vi "log file viewer.vi"() -> ()   [LabVIEW 2020]
uses:
  <vilib>/Utility/sysdir.llb/System Directory Type.ctl
  <vilib>/addons/_JKI Toolkits/State Machine/_JKI_lib_State_Machine.llb/Select State(s)_err__jki_lib_state_machine.vi
  <vilib>/regexp/Match Regular Expression.xnode
  <vilib>/JDP Science/JSONtext/JSONtext.lvlib
panel:
  in  "Open File":bool
  in  "refresh":bool
  in  "Log Files":i32(listbox)
  out "message":string
  in  "timestamp":i32(listbox)
  in  "Exit":bool
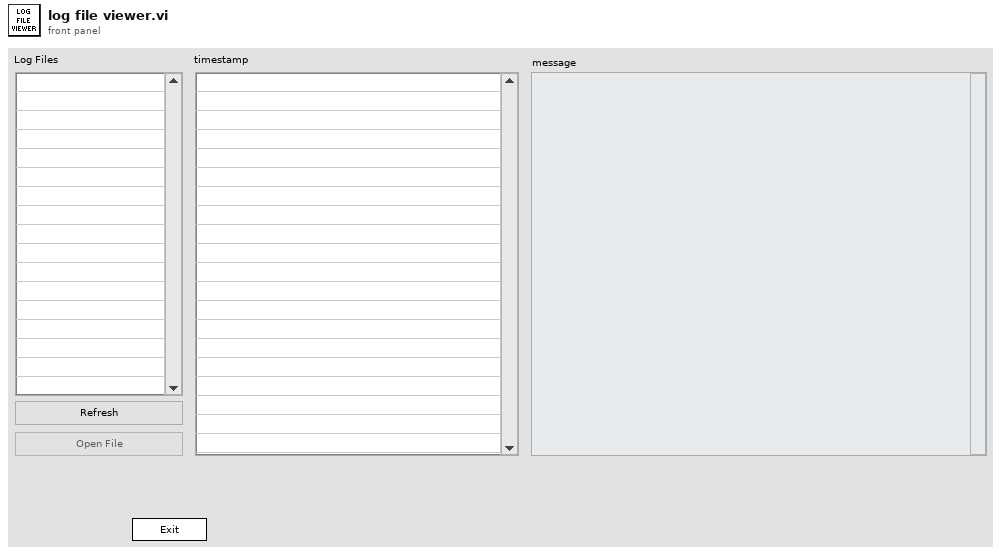
[diagram p1: front panel]
types:
  T1 = enum8{"Enabled", "Disabled", "Disabled and Grayed Out"}
  T2 = enum32{"Invalid", "Standard", "Closed", "Hidden", "Minimized", "Maximized"}
  T3 = enum32{"invalid app kind", "Development System", "Run Time System", "Student Edition", "Embedded LabVIEW", "Evaluation", "Custom"}
  T4 = cluster{"Core":cluster{"Current VI Reference":refnum<vi>, "Close Panel on Exit?":bool}, "log file":path, "elements":string[], "Log Directory":path}
  T5 = typedef "System Directory Type.ctl" = i32
  T6 = cluster{"Current VI Reference":refnum<vi>, "Close Panel on Exit?":bool}
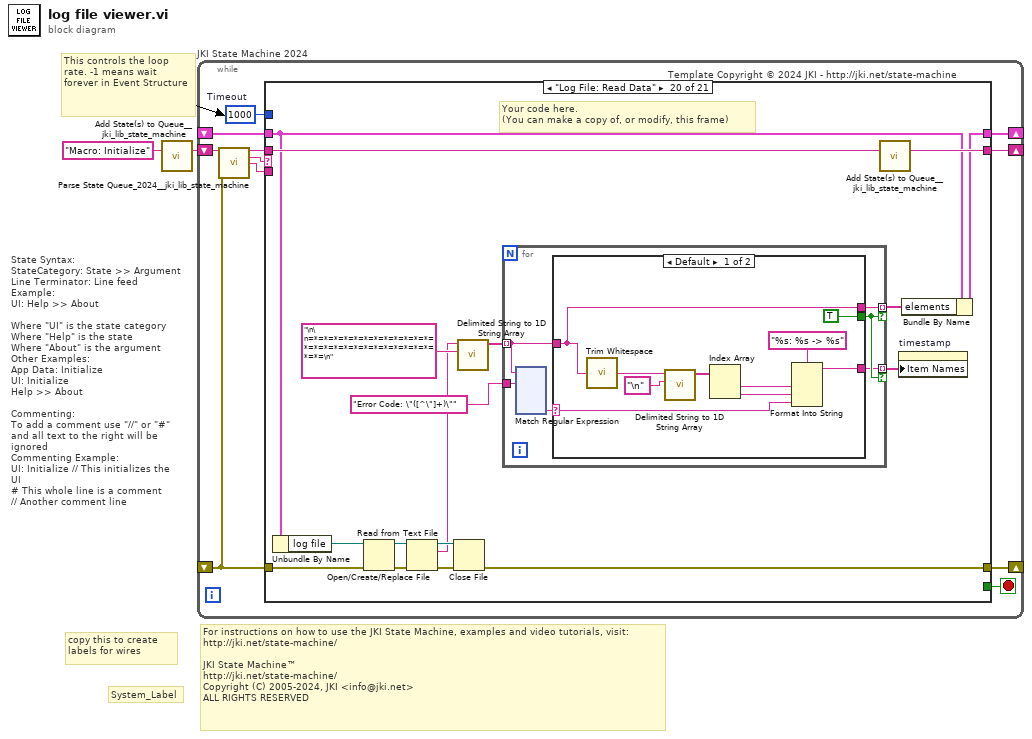
[diagram p0: block diagram]
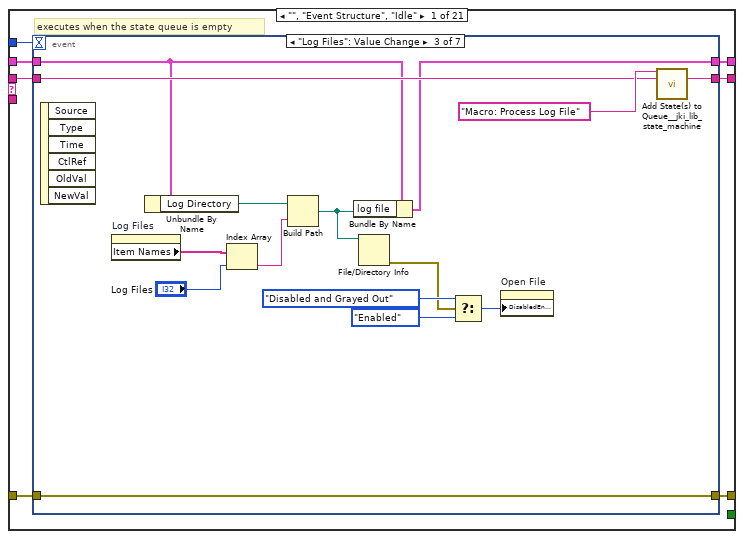
[diagram p2: hidden frame]
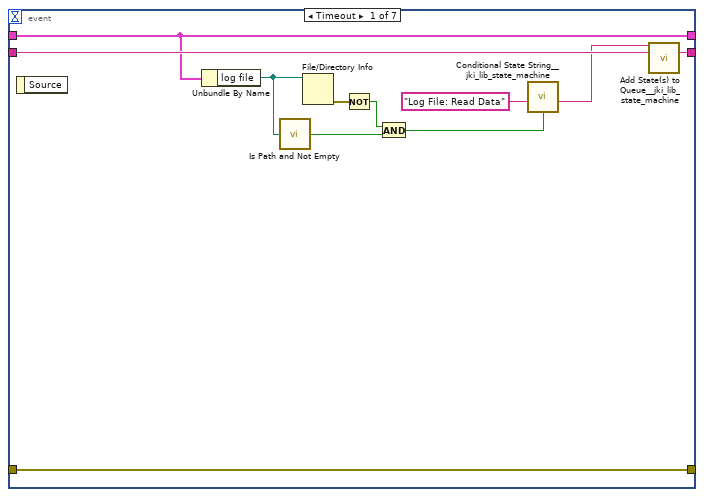
[diagram p3: hidden frame]
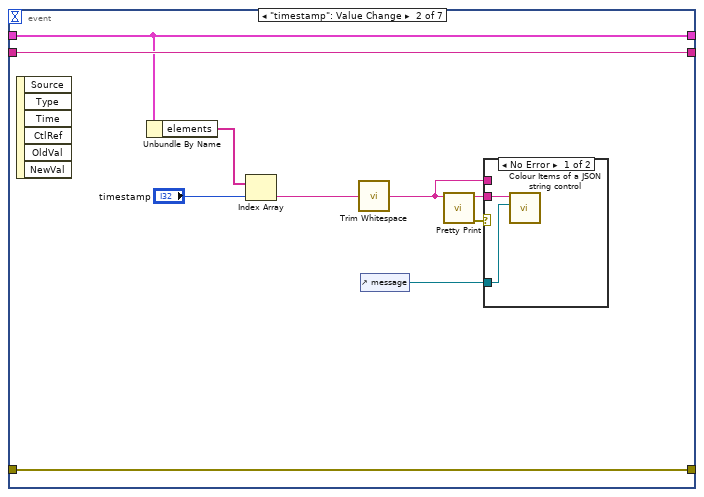
[diagram p4: hidden frame]
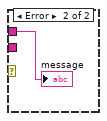
[diagram p5: hidden frame]
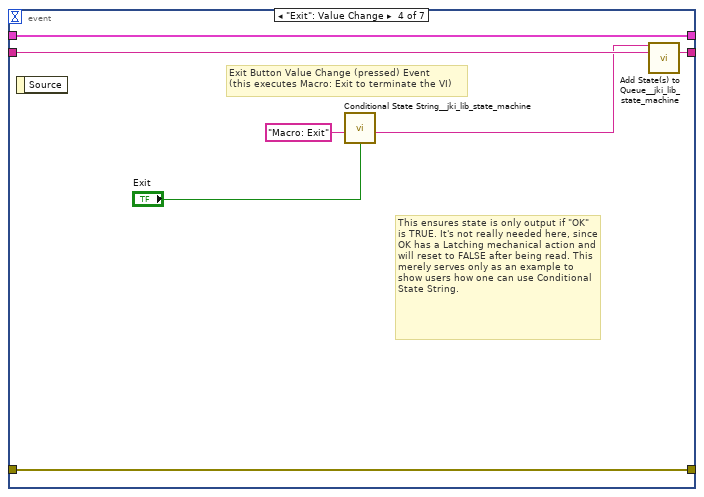
[diagram p6: hidden frame]
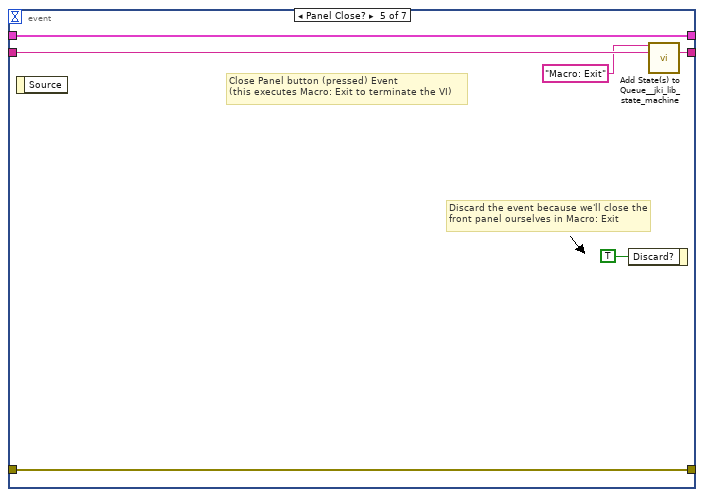
[diagram p7: hidden frame]
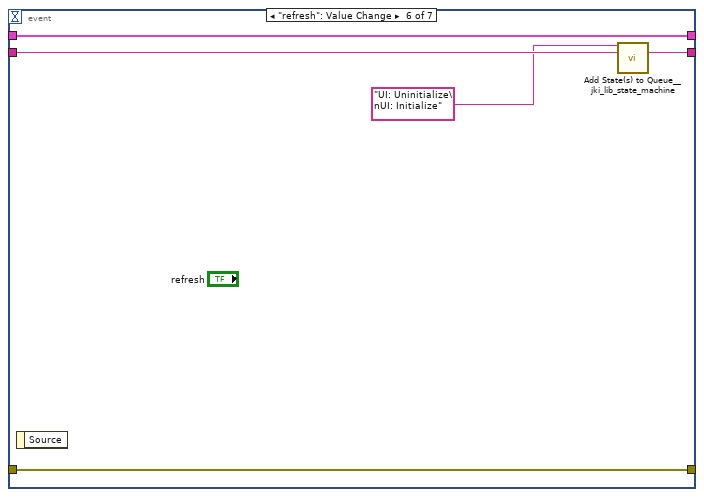
[diagram p8: hidden frame]
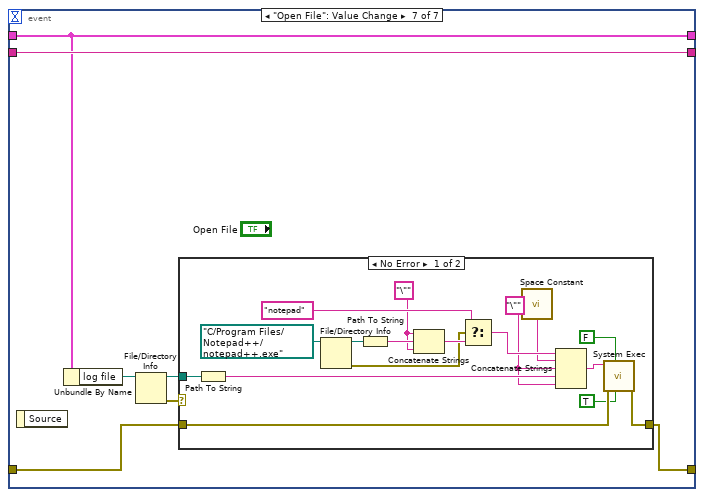
[diagram p9: hidden frame]
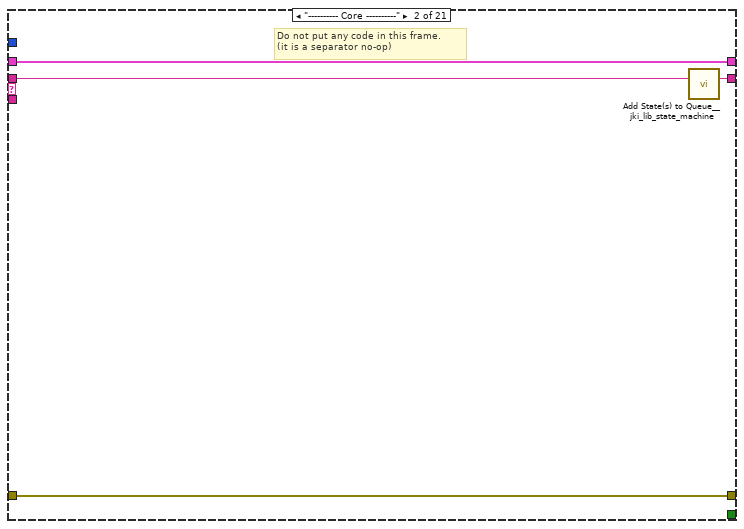
[diagram p11: hidden frame]
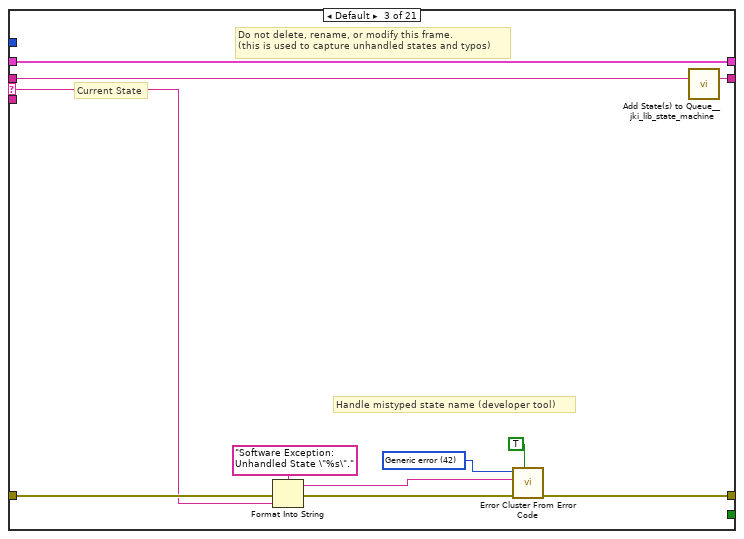
[diagram p12: hidden frame]
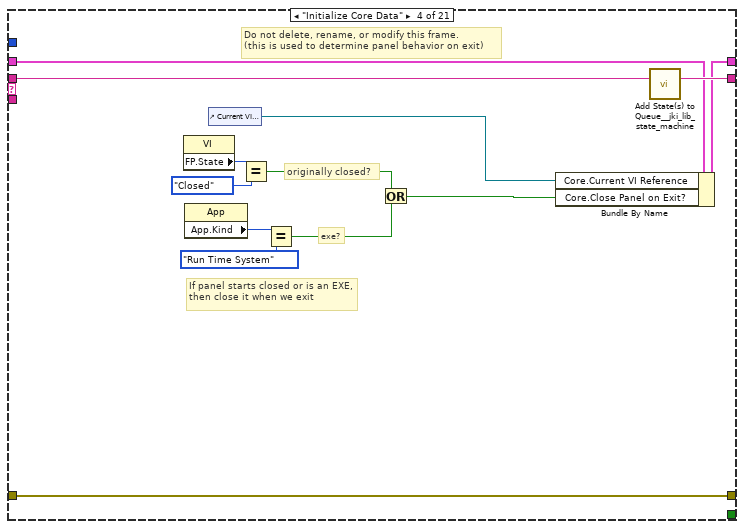
[diagram p13: hidden frame]
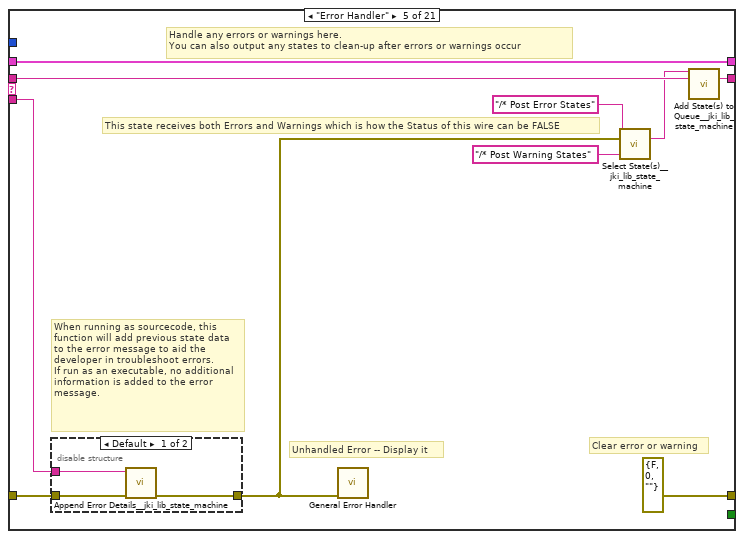
[diagram p14: hidden frame]
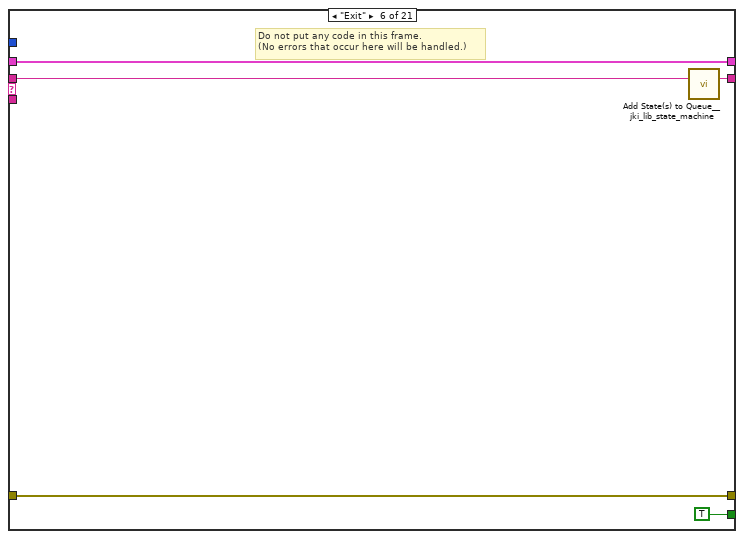
[diagram p16: hidden frame]
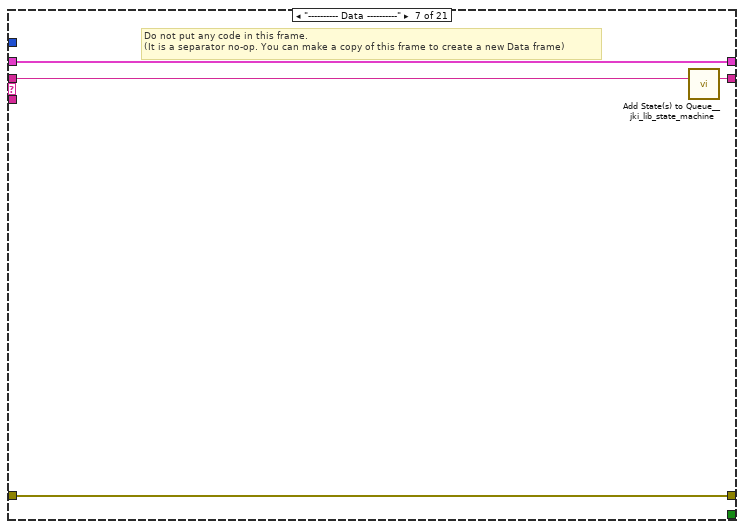
[diagram p17: hidden frame]
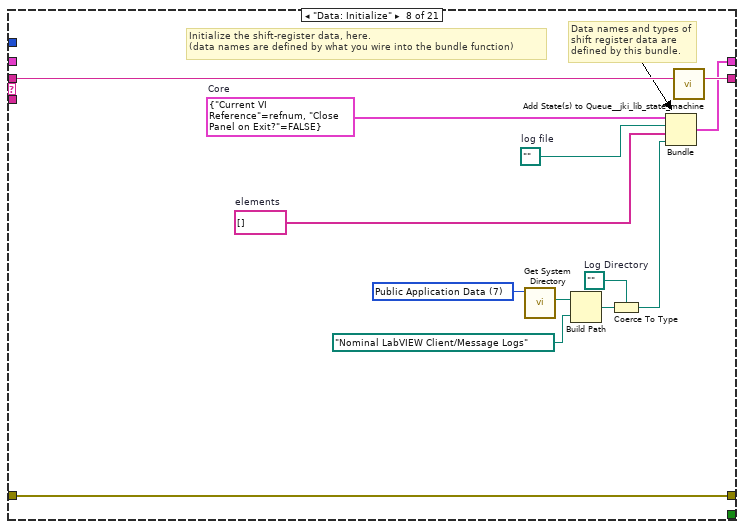
[diagram p18: hidden frame]
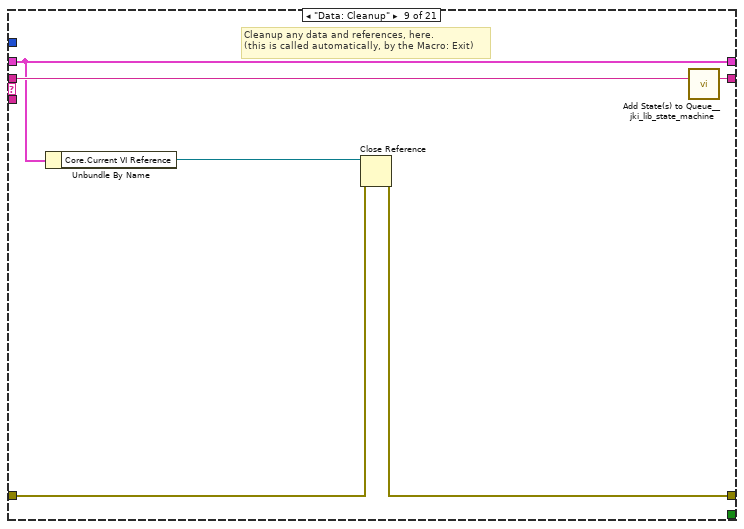
[diagram p19: hidden frame]
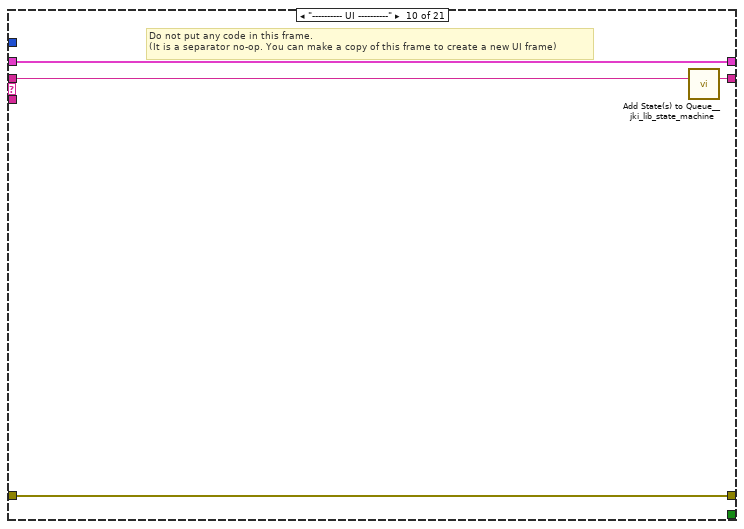
[diagram p20: hidden frame]
diagram:
  # "For instructions on how to use the JKI State Machine, examples and video tutorials, visit:\nhttp://jki.net/state-machine/\n\nJKI State Machine™\nhttp://jki.net/state-machine/\nCopyright (C) 2005-2024, JKI <info@jki.net>\nALL RIGHTS RESERVED"
  # "State Syntax:\nStateCategory: State >> Argument\nLine Terminator: Line feed\nExample:\nUI: Help >> About\n\nWhere \"UI\" is the state category\nWhere \"Help\" is the state\nWhere \"About\" is the argument\nOther Examples:\nApp Data: Initialize\nUI: Initialize\nHelp >> About\n\nCommenting:\nTo add a comment use \"//\" or \"#\" and all text to the right will be ignored\nCommenting Example:\nUI: Initialize // This initializes the UI\n# This whole line is a comment\n// Another comment line"
  # "copy this to create labels for wires"
  # "This controls the loop rate. -1 means wait forever in Event Structure"
  # "System_Label"
  n1 = call <vilib>:"Add State(s) to Queue__jki_lib_state_machine.vi"("State(s) in (\"\")"="Macro: Initialize") -> ("States Out"=w2:string)  [unwired: 14 in]
  n2 = while "JKI State Machine 2024" {
    shift-right: [w6] -> _
    shift-left: _ -> [w5]
    shift-right: [w9] -> _
    shift-left: _ -> [w3]
    shift-right: [w8] -> _
    shift-left: w2 -> [w10]
    stop <- w7 stop-if-true
    w4 = 1000  # Timeout
    # "Template Copyright © 2024 JKI - http://jki.net/state-machine"
    n3 = call <vilib>:"Parse State Queue_2024__jki_lib_state_machine.vi"("State Queue"=w10, "Error In (no error)"=w3) -> ("Remaining States"=w12:string, "Current State"=w13:string, "Arguments"=w11:string)  [unwired: 11 in]
    n4 = case shown="\"Log File: Read Data\"" w13 {
      selector: w13 -> [_ _ w107 _ _ _ _ _ _ _ _ _ _ _ _ _ _ _ _ _ _]
      tunnel: w12 -> [w20 w106 w111 w130 w140 w149 w153 w166 w172 w176 w184 w186 w197 w208 w277 w282 w291 w296 w300 w317 w466]
      tunnel: w11 -> [_ _ _ _ w135 _ _ _ _ _ _ _ w192 w202 _ _ _ _ _ _ _]
      tunnel: w5 -> [w18 w103 w109 w123 w137 w147 w150 _ w167 w173 w180 w190 w195 w204 w274 w279 w289 w294 w297 w304 w463]
      tunnel: [w17 w104 w113 w127 errorcluster {"status"=FALSE, "code"=0, "source"=""} ("error out") w146 w151 w163 w168 w174 w182 w189 w193 w205 w275 w280 w286 w293 w298 w310 w464] -> w9
      tunnel: w3 -> [w14 w104 w112 w127 w136 w146 w151 w163 w169 w174 w182 w189 w194 w206 w275 w280 w286 w293 w298 w309 w464]
      tunnel: [w19 w105 w110 w129 w139 w148 w152 w165 w171 w175 w183 w191 w196 w207 w276 w281 w290 w295 w299 w316 w465] -> w8
      tunnel: [_ _ _ _ _ TRUE _ _ _ _ _ _ _ _ _ _ _ _ _ _ _] -> w7
      tunnel: [w16 w103 w109 w128 w137 w147 w150 w164 w167 w173 w180 w190 w195 w204 w274 w279 w289 w294 w297 w303 w463] -> w6
      tunnel: w4 -> [w15 _ _ _ _ _ _ _ _ _ _ _ _ _ _ _ _ _ _ _ _]
      frame "", "Event Structure", "Idle" {
        # "executes when the state queue is empty"
        n5 = event shown="[2] \"Log Files\": Value Change" {
          selector: _ -> [_ _ _ _ _ _ _]
          dyn-events: _ -> [_ _ _ _ _ _ _]
          timeout: w15 -> [_ _ _ _ _ _ _]
          tunnel: w20 -> [w31 w41 w57 w66 w72 w75 w84]
          tunnel: [w30 w41 w56 w65 w71 w76 w84] -> w19
          tunnel: w18 -> [w28 w40 w51 w63 w69 w77 w83]
          tunnel: [w29 w33 w59 w64 w70 w74 w78] -> w17
          tunnel: w14 -> [w29 w33 w59 w64 w70 w74 w79]
          tunnel: [w28 w40 w50 w63 w69 w77 w83] -> w16
          event Timeout {
            n6 = event-data() -> ()  [unwired: 1 in, 1 out]
            n7 = Unbundle By Name(w28) -> ("log file"=w26:path)
            n8 = call <vilib>:"Is Path and Not Empty.vi"("path"=w26) -> ("Is Path and Not Empty?"=w25:bool)  [unwired: 4 in]
            n9 = File/Directory Info(path=w26) -> (error out=w27:errorcluster)  [unwired: 1 in, 6 out]
            n10 = Not(x=w27) -> (.not. x?=w24:bool)
            n11 = And(x=w24, y=w25) -> (x .and. y?=w22:bool)
            n12 = call <vilib>:"Conditional State String__jki_lib_state_machine.vi"("Do State(s)?"=w22, "State"="Log File: Read Data") -> ("State Out"=w23:string)  [unwired: 7 in]
            n13 = call <vilib>:"Add State(s) to Queue__jki_lib_state_machine.vi"("State(s) in Front (\"\")"=w23, "State(s) in (\"\")"=w31) -> ("States Out"=w30:string)  [unwired: 13 in]
          }
          event "timestamp": Value Change {
            n14 = event-data() -> ()  [unwired: 1 in, 6 out]
            n15 = Unbundle By Name(w40) -> ("elements"=w39:string[])
            n16 = Index Array(array=w39, index="timestamp") -> (element=w32:string)
            n17 = call <vilib>:"Trim Whitespace.vi"("string"=w32) -> ("trimmed string"=w34:string)  [unwired: 1 in]
            n18 = control-ref of="message"() -> (w37:refnum<vi>)
            n19 = call <vilib>:"Pretty Print.vi"("JSON"=w34) -> ("error out"=w35:errorcluster, "<JSON>"=w36:string)  [unwired: 8 in, 1 out]
            n20 = case shown="No Error" w35 {
              tunnel: w37 -> [w43 _]
              tunnel: w36 -> [w42 _]
              tunnel: w34 -> [_ w44]
              frame No Error {
                n21 = call <vilib>:"Colour Items of a JSON string control.vi"("String Control"=w43, "JSON"=w42) -> ()  [unwired: 9 in, 1 out]
              }
              frame Error {
                "message" <- w44
              }
            }
          }
          event "Log Files": Value Change {
            n22 = event-data() -> ()  [unwired: 1 in, 6 out]
            n23 = property on="Log Files" class="LstBox (strict)"() -> ("Item Names"=w54:string[])  [unwired: 2 in, 2 out]
            n24 = Unbundle By Name(w51) -> ("Log Directory"=w55:path)
            n25 = Index Array(array=w54, index="Log Files") -> (element=w52:string)
            n26 = Build Path(base path=w55, name or relative path=w52) -> (appended path=w46:path)
            n27 = Bundle By Name(cluster=w51, "log file"=w46) -> (w50:T4)
            n28 = File/Directory Info(path=w46) -> (error out=w45:errorcluster)  [unwired: 1 in, 6 out]
            n29 = Select(t=T1."Disabled and Grayed Out" ("Disabled"), s=w45, f=T1."Enabled" ("Disabled")) -> (s? t:f=w47:T1)
            n30 = property on="Open File" class="Bool"("DisabledEnum"=w47) -> ()  [unwired: 2 in, 2 out]
            n31 = call <vilib>:"Add State(s) to Queue__jki_lib_state_machine.vi"("State(s) in Front (\"\")"="Macro: Process Log File" ("string"), "State(s) in (\"\")"=w57) -> ("States Out"=w56:string)  [unwired: 13 in]
          }
          event "Exit": Value Change {
            # "This ensures state is only output if \"OK\" is TRUE. It's not really needed here, since OK has a Latching mechanical action and will reset to FALSE after being read. This merely serves only as an example to show users how one can use Conditional State String."
            # "Exit Button Value Change (pressed) Event\n(this executes Macro: Exit to terminate the VI)"
            n32 = event-data() -> ()  [unwired: 1 in, 1 out]
            n33 = call <vilib>:"Conditional State String__jki_lib_state_machine.vi"("Do State(s)?"="Exit", "State"="Macro: Exit") -> ("State Out"=w60:string)  [unwired: 7 in]
            n34 = call <vilib>:"Add State(s) to Queue__jki_lib_state_machine.vi"("State(s) in Front (\"\")"=w60, "State(s) in (\"\")"=w66) -> ("States Out"=w65:string)  [unwired: 13 in]
          }
          event Panel Close? {
            # "Discard the event because we'll close the front panel ourselves in Macro: Exit"
            # "Close Panel button (pressed) Event\n(this executes Macro: Exit to terminate the VI)"
            n35 = event-data() -> ()  [unwired: 1 in, 1 out]
            n36 = event-data("Discard?"=TRUE) -> ()  [unwired: 1 in, 1 out]
            n37 = call <vilib>:"Add State(s) to Queue__jki_lib_state_machine.vi"("State(s) in Front (\"\")"="Macro: Exit", "State(s) in (\"\")"=w72) -> ("States Out"=w71:string)  [unwired: 13 in]
          }
          event "refresh": Value Change {
            n38 = event-data() -> ()  [unwired: 1 in, 1 out]
            n39 = call <vilib>:"Add State(s) to Queue__jki_lib_state_machine.vi"("State(s) in Front (\"\")"="UI: Uninitialize\nUI: Initialize" ("State(s) in Front (\"\")"), "State(s) in (\"\")"=w75) -> ("States Out"=w76:string)  [unwired: 13 in]
          }
          event "Open File": Value Change {
            n40 = event-data() -> ()  [unwired: 1 in, 1 out]
            n41 = Unbundle By Name(w83) -> ("log file"=w82:path)
            n42 = File/Directory Info(path=w82) -> (path out=w80:path, error out=w81:errorcluster)  [unwired: 1 in, 5 out]
            n43 = case shown="No Error" w81 {
              tunnel: w80 -> [w98 _]
              tunnel: w79 -> [w92 w102]
              tunnel: [w91 w102] -> w78
              frame No Error {
                w88 = "\"" ("string")
                w95 = "\"" ("string")
                n44 = Path To String(path=w98) -> (string=w96:string)
                n45 = File/Directory Info(path=path "C:/Program Files/Notepad++/notepad++.exe") -> (path out=w101:path, error out=w86:errorcluster)  [unwired: 1 in, 5 out]
                n46 = Path To String(path=w101) -> (string=w89:string)
                n47 = Concatenate Strings(w88, w89, w88) -> (w87:string)
                n48 = Select(t="notepad", s=w86, f=w87) -> (s? t:f=w97:string)
                n49 = call <vilib>:"Space Constant.vi"() -> ("String"=w94:string)
                n50 = Concatenate Strings(w97, w94, w95, w96, w95) -> (w93:string)
                n51 = call <vilib>:"System Exec.vi"("run minimized? (F)"=TRUE, "wait until completion? (T)"=FALSE, "error in (no error)"=w92, "command line"=w93) -> ("error out"=w91:errorcluster)  [unwired: 4 in, 3 out]
              }
              frame Error {
              }
            }
          }
        }
      }
      frame "---------- Core ----------" {
        # "Do not put any code in this frame.\n(it is a separator no-op)"
        n52 = call <vilib>:"Add State(s) to Queue__jki_lib_state_machine.vi"("State(s) in (\"\")"=w106) -> ("States Out"=w105:string)  [unwired: 14 in]
      }
      frame Default {
        w116 = 42 items=["No error", "Argument error", "Memory is full", "Out of zone", "End of file", "File already open", "Generic file I/O error", "File not found", "File permission error", "Disk is full", "Duplicate path", "Too many files open", "System feature not enabled", "Resource file not found", "Cannot add resource", "Resource not found", "Image not found", "Image memory error", "Pen does not exist", "Config type invalid", "Config token not found", "Config parse error", "Config memory error", "Bad external code format", "Bad external code offset", "External code not present", "Null window", "Destroy window error", "Null menu", "Print aborted", "Bad print record", "Print driver error", "Windows error during printing", "Memory error during printing", "Print dialog error", "Generic print error", "Invalid device refnum", "Device not found", "Device parameter error", "Device unit error", "Cannot open device", "Device call aborted", "Generic error", "Cancelled by user", "Object ID too low", "Object ID too high", "Object not in heap", "Unknown heap", "Unknown object (invalid DefProc)", "Unknown object (DefProc not in table)", "Message out of range", "Invalid (null) method", "Unknown message", "Manager call not supported", "Bad address", "Network operation in progress", "Network operation timed out", "Connection is busy", "Network attribute not supported", "Network error", "Address in use", "System out of memory", "Connection aborted", "Connection refused", "Not connected", "Already connected", "Connection closed", "Initialization error (interapplication manager)", "Bad occurrence", "Wait on unbound occurrence handler", "Occurrence queue overflow", "Datalog type conflict", "Unused", "Unrecognized type (interapplication manager)", "Memory corrupt", "Failed to make temporary DLL", "Old CIN version", "Drag socket not found", "Failed to load drop-object", "Failed to register OLE object", "Failed to release OLE object", "Format specifier type mismatch", "Unknown format specifier", "Too few format specifiers", "Too many format specifiers", "Scan failed", "Newer CIN version", "Error converting to variant", "Runtime menu error", "Password tampered", "Variant attribute not found", "Incompatible variant data type", "Event data is not available", "Event Store is not present", "Occurrence is not found", "Event Queue is not created", "Event info is not available", "Refnum passed is NULL", "Error retrieving Class GUID", "Error retrieving CoClass GUID", "Error retrieving TypeLib GUID.", "Bad built application magic bytes.", "Specific driver is different from the specific driver associated with the Logical Name.", "There is no session opened to the class driver.", "Max Error", "MAX - Error with config objects", "MAX - Error loading configuration", "MAX - Group not supported"]
        # "Current State"
        # "Do not delete, rename, or modify this frame.\n(this is used to capture unhandled states and typos)"
        # "Handle mistyped state name (developer tool)"
        n53 = Format Into String(format string="Software Exception: Unhandled State \"%s\"." ("message"), error in=w112, w107) -> (resulting string=w115:string, error out=w114:errorcluster)  [unwired: 1 in]
        n54 = call <vilib>:"Error Cluster From Error Code.vi"("show call chain? (False)"=TRUE, "error in (no error)"=w114, "error message (\"\")"=w115, "error code (0)"=w116) -> ("error out"=w113:errorcluster)  [unwired: 5 in]
        n55 = call <vilib>:"Add State(s) to Queue__jki_lib_state_machine.vi"("State(s) in (\"\")"=w111) -> ("States Out"=w110:string)  [unwired: 14 in]
      }
      frame "Initialize Core Data" {
        # "Do not delete, rename, or modify this frame.\n(this is used to determine panel behavior on exit)"
        # "originally closed?"
        # "exe?"
        # "If panel starts closed or is an EXE, then close it when we exit"
        n56 = property class="VI"() -> ("FP.State"=w120:T2)  [unwired: 2 in, 2 out]
        n57 = property class="App"() -> ("App.Kind"=w126:T3)  [unwired: 2 in, 2 out]
        n58 = control-ref of="Current VI Reference"() -> (w121:refnum<vi>)
        n59 = Equal?(x=w120, y=T2."Closed" ("Front Panel Window:State")) -> (x = y?=w118:bool)
        n60 = Equal?(x=w126, y=T3."Run Time System" ("Application:Kind")) -> (x = y?=w124:bool)
        n61 = Or(x=w118, y=w124) -> (x .or. y?=w122:bool)
        n62 = Bundle By Name(cluster=w123, "Core.Current VI Reference"=w121, "Core.Close Panel on Exit?"=w122) -> (w128:T4)
        n63 = call <vilib>:"Add State(s) to Queue__jki_lib_state_machine.vi"("State(s) in (\"\")"=w130) -> ("States Out"=w129:string)  [unwired: 14 in]
      }
      frame "Error Handler" {
        # "When running as sourcecode, this function will add previous state data to the error message to aid the developer in troubleshoot errors.\nIf run as an executable, no additional information is added to the error message."
        # "This state receives both Errors and Warnings which is how the Status of this wire can be FALSE"
        # "Unhandled Error -- Display it"
        # "Handle any errors or warnings here.\nYou can also output any states to clean-up after errors or warnings occur"
        # "Clear error or warning"
        n64 = disable-structure shown="Default" {
          disable-tunnel: w136 -> [w143 w144]
          disable-tunnel: w135 -> [w142 _]
          disable-tunnel: [w141 w144] -> w134
          frame condition #0 (active) {
            n65 = call <vilib>:"Append Error Details__jki_lib_state_machine.vi"("error in (no error)"=w143, "Previous State and Argument(s)"=w142) -> ("error out"=w141:errorcluster)  [unwired: 9 in]
          }
          frame condition #1 {
          }
        }
        n66 = call <vilib>:"General Error Handler.vi"("error in (no error)"=w134) -> ()  [unwired: 10 in, 5 out]
        n67 = call-poly <vilib>:"Select State(s)__jki_lib_state_machine.vi"("State(s) if True (\"\")"="/* Post Error States", "Select"=w134, "State(s) if False (\"\")"="/* Post Warning States") -> ("States Out"=w132:string)  [unwired: 12 in]
        n68 = call <vilib>:"Add State(s) to Queue__jki_lib_state_machine.vi"("State(s) in Front (\"\")"=w132, "State(s) in (\"\")"=w140) -> ("States Out"=w139:string)  [unwired: 13 in]
      }
      frame "Exit" {
        # "Do not put any code in this frame.\n(No errors that occur here will be handled.)"
        n69 = call <vilib>:"Add State(s) to Queue__jki_lib_state_machine.vi"("State(s) in (\"\")"=w149) -> ("States Out"=w148:string)  [unwired: 14 in]
      }
      frame "---------- Data ----------" {
        # "Do not put any code in this frame.\n(It is a separator no-op. You can make a copy of this frame to create a new Data frame)"
        n70 = call <vilib>:"Add State(s) to Queue__jki_lib_state_machine.vi"("State(s) in (\"\")"=w153) -> ("States Out"=w152:string)  [unwired: 14 in]
      }
      frame "Data: Initialize" {
        w154 = path ""  # Log Directory
        w159 = T5 7 items=["User Home"=0, "User Desktop"=1, "User Documents"=2, "User Application Data"=3, "User Preferences"=4, "User Temporary"=5, "Public Documents"=6, "Public Application Data"=7, "Public Preferences"=8, "Public Cache"=13, "System Core Libraries"=9, "System Installed Libraries"=10, "Application Files"=11, "Boot Volume Root"=12] ("system directory type")
        w160 = string[] []  # elements
        w161 = path ""  # log file
        w162 = T6 {"Current VI Reference"=refnum, "Close Panel on Exit?"=FALSE}  # Core
        # "Data names and types of shift register data are defined by this bundle."
        # "Initialize the shift-register data, here.\n(data names are defined by what you wire into the bundle function)"
        n71 = call <vilib>:"Get System Directory.vi"("system directory type"=w159) -> ("system directory"=w158:path)  [unwired: 10 in]
        n72 = Build Path(base path=w158, name or relative path=path "Nominal LabVIEW Client/Message Logs") -> (appended path=w156:path)
        n73 = Coerce To Type(0:w156, 1:w154) -> (2:w155:path)
        n74 = Bundle("Core"=w162, "log file"=w161, "elements"=w160, "Log Directory"=w155) -> (w164:T4)  [unwired: 1 in]
        n75 = call <vilib>:"Add State(s) to Queue__jki_lib_state_machine.vi"("State(s) in (\"\")"=w166) -> ("States Out"=w165:string)  [unwired: 14 in]
      }
      frame "Data: Cleanup" {
        # "Cleanup any data and references, here.\n(this is called automatically, by the Macro: Exit)"
        n76 = Unbundle By Name(w167) -> ("Core.Current VI Reference"=w170:refnum<vi>)
        n77 = Close Reference(reference=w170, error in (no error)=w169) -> (error out=w168:errorcluster)
        n78 = call <vilib>:"Add State(s) to Queue__jki_lib_state_machine.vi"("State(s) in (\"\")"=w172) -> ("States Out"=w171:string)  [unwired: 14 in]
      }
      frame "---------- UI ----------" {
        # "Do not put any code in this frame.\n(It is a separator no-op. You can make a copy of this frame to create a new UI frame)"
        n79 = call <vilib>:"Add State(s) to Queue__jki_lib_state_machine.vi"("State(s) in (\"\")"=w176) -> ("States Out"=w175:string)  [unwired: 14 in]
      }
      frame "UI: Initialize" {
        w178 = 0 ("Top Row")
        # "Initialize the User Interface, here.\n(this is called automatically, by the Macro: Initialize)"
        n80 = Unbundle By Name(w180) -> ("Log Directory"=w179:path)
        n81 = List Folder(path=w179) -> (filenames=w181:string[])  [unwired: 3 in, 3 out]
        n82 = property on="Open File" class="Bool"("DisabledEnum"=T1."Disabled and Grayed Out" ("Disabled")) -> ()  [unwired: 2 in, 2 out]
        n83 = property on="Log Files" class="LstBox (strict)"("Item Names"=w181, "Top Row"=w178) -> ()  [unwired: 2 in, 2 out]
        n84 = property on="timestamp" class="LstBox (strict)"("Top Row"=w178) -> ()  [unwired: 2 in, 2 out]
        n85 = call <vilib>:"Add State(s) to Queue__jki_lib_state_machine.vi"("State(s) in (\"\")"=w184) -> ("States Out"=w183:string)  [unwired: 14 in]
      }
      frame "UI: Uninitialize" {
        w188 = string[] [] ("Item Names")
        # "Cleanup the User Interface, here.\n(this is called automatically, by the Macro: Exit)"
        n86 = local write "message"("") -> ()
        n87 = property on="Log Files" class="LstBox (strict)"("Item Names"=w188) -> ()  [unwired: 2 in, 2 out]
        n88 = property on="timestamp" class="LstBox (strict)"("Item Names"=w188) -> ()  [unwired: 2 in, 2 out]
        n89 = property on="Open File" class="Bool"("DisabledEnum"=T1."Disabled and Grayed Out" ("Disabled")) -> ()  [unwired: 2 in, 2 out]
        n90 = call <vilib>:"Add State(s) to Queue__jki_lib_state_machine.vi"("State(s) in (\"\")"=w186) -> ("States Out"=w191:string)  [unwired: 14 in]
      }
      frame "UI: Cursor Set" {
        # "Argument"
        # "Set and Unset Cursor Busy.\n(Usage: \"UI: Cursor Set >> Busy|Idle\")"
        n91 = case shown="\"Idle\", Default" w192 {
          tunnel: w194 -> [w199 w201]
          tunnel: [w198 w200] -> w193
          frame "Idle", Default {
            n92 = call <vilib>:"Unset Busy.vi"("error in (no error)"=w199) -> ("error out"=w198:errorcluster)  [unwired: 10 in]
          }
          frame "Busy" {
            n93 = call <vilib>:"Set Busy.vi"("error in (no error)"=w201) -> ("error out"=w200:errorcluster)  [unwired: 9 in, 1 out]
          }
        }
        n94 = call <vilib>:"Add State(s) to Queue__jki_lib_state_machine.vi"("State(s) in (\"\")"=w197) -> ("States Out"=w196:string)  [unwired: 14 in]
      }
      frame "UI: Front Panel State" {
        # "Argument"
        # "Set Front Panel Open or Closed\n(Usage: \"UI: Front Panel State >> Open|Close\")"
        n95 = Unbundle By Name(w204) -> ("Core.Current VI Reference"=w203:refnum<vi>)
        n96 = case shown="\"Minimize\", \"Minimized\"" w202 {
          tunnel: w206 -> [w214 w229 w240 w253 w266]
          tunnel: [w216 w230 w242 w255 w268] -> w205
          tunnel: w203 -> [w215 w227 w241 w254 w267]
          frame "Open", "Standard", Default {
            w209 = T2."Standard" ("State")
            n97 = property class="VI"(reference=w215, error in=w214) -> (reference out=w212:refnum<vi>, error out=w213:errorcluster, "FP.State"=w211:T2)
            n98 = Not Equal?(x=w211, y=w209) -> (x != y?=w210:bool)
            n99 = case shown="True" w210 {
              tunnel: [w220 w222] -> w216
              tunnel: w213 -> [w219 w222]
              tunnel: w212 -> [w218 _]
              tunnel: w209 -> [w217 _]
              frame True {
                n100 = invoke class="VI" method="FP.Open"(reference=w218, error in=w219, "Activate"=TRUE, "State"=w217) -> (error out=w220:errorcluster)  [unwired: 1 in, 4 out]
              }
              frame False {
              }
            }
          }
          frame "Close", "Closed" {
            n101 = property class="VI"(reference=w227, error in=w229) -> (reference out=w226:refnum<vi>, error out=w228:errorcluster, "FP.State"=w224:T2)
            n102 = Not Equal?(x=w224, y=T2."Closed" ("Front Panel Window:State")) -> (x != y?=w223:bool)
            n103 = case shown="True" w223 {
              tunnel: [w231 w234] -> w230
              tunnel: w228 -> [w231 w233]
              tunnel: w226 -> [_ w232]
              frame False {
              }
              frame True {
                n104 = invoke class="VI" method="FP.Close"(reference=w232, error in=w233) -> (error out=w234:errorcluster)  [unwired: 1 in, 2 out]
              }
            }
          }
          frame "Hidden", "Hide" {
            w235 = T2."Hidden" ("State")
            n105 = property class="VI"(reference=w241, error in=w240) -> (reference out=w238:refnum<vi>, error out=w239:errorcluster, "FP.State"=w237:T2)
            n106 = Not Equal?(x=w237, y=w235) -> (x != y?=w236:bool)
            n107 = case shown="True" w236 {
              tunnel: [w246 w247] -> w242
              tunnel: w239 -> [w245 w247]
              tunnel: w238 -> [w244 _]
              tunnel: w235 -> [w243 _]
              frame True {
                n108 = invoke class="VI" method="FP.Open"(reference=w244, error in=w245, "State"=w243) -> (error out=w246:errorcluster)  [unwired: 2 in, 4 out]
              }
              frame False {
              }
            }
          }
          frame "Minimize", "Minimized" {
            w248 = T2."Minimized" ("State")
            n109 = property class="VI"(reference=w254, error in=w253) -> (reference out=w251:refnum<vi>, error out=w252:errorcluster, "FP.State"=w250:T2)
            n110 = Not Equal?(x=w250, y=w248) -> (x != y?=w249:bool)
            n111 = case shown="True" w249 {
              tunnel: [w259 w260] -> w255
              tunnel: w252 -> [w258 w260]
              tunnel: w251 -> [w257 _]
              tunnel: w248 -> [w256 _]
              frame True {
                n112 = invoke class="VI" method="FP.Open"(reference=w257, error in=w258, "State"=w256) -> (error out=w259:errorcluster)  [unwired: 2 in, 4 out]
              }
              frame False {
              }
            }
          }
          frame "Maximize", "Maximized" {
            w261 = T2."Maximized" ("State")
            n113 = property class="VI"(reference=w267, error in=w266) -> (reference out=w264:refnum<vi>, error out=w265:errorcluster, "FP.State"=w263:T2)
            n114 = Not Equal?(x=w263, y=w261) -> (x != y?=w262:bool)
            n115 = case shown="True" w262 {
              tunnel: [w272 w273] -> w268
              tunnel: w265 -> [w271 w273]
              tunnel: w264 -> [w270 _]
              tunnel: w261 -> [w269 _]
              frame True {
                n116 = invoke class="VI" method="FP.Open"(reference=w270, error in=w271, "State"=w269) -> (error out=w272:errorcluster)  [unwired: 2 in, 4 out]
              }
              frame False {
              }
            }
          }
        }
        n117 = call <vilib>:"Add State(s) to Queue__jki_lib_state_machine.vi"("State(s) in (\"\")"=w208) -> ("States Out"=w207:string)  [unwired: 14 in]
      }
      frame "---------- Macro ----------" {
        # "Do not put any code in this frame.\n(It is a separator no-op. You can make a copy of this frame to create a new Macro frame)"
        n118 = call <vilib>:"Add State(s) to Queue__jki_lib_state_machine.vi"("State(s) in (\"\")"=w277) -> ("States Out"=w276:string)  [unwired: 14 in]
      }
      frame "Macro: Initialize" {
        w278 = "Data: Initialize\nInitialize Core Data\nUI: Initialize\nUI: Front Panel State >> Open"  # Data: Initialize Initialize Core Data UI: Initialize UI: Front Panel State >> Open
        # "Initialization Macro\n(This is called once, when the VI starts)"
        n119 = call <vilib>:"Add State(s) to Queue__jki_lib_state_machine.vi"("State(s) in Front (\"\")"=w278, "State(s) in (\"\")"=w282) -> ("States Out"=w281:string)  [unwired: 13 in]
      }
      frame "Macro: Exit" {
        # "Exit Macro\n(This is called once, when the VI exits)"
        n120 = Unbundle By Name(w289) -> ("Core.Close Panel on Exit?"=w284:bool)
        n121 = call <vilib>:"Conditional State String__jki_lib_state_machine.vi"("Do State(s)?"=w284, "State"="UI: Front Panel State >> Close") -> ("State Out"=w283:string)  [unwired: 7 in]
        n122 = call <vilib>:"Add State(s) to Queue__jki_lib_state_machine.vi"("State(s) in (\"\")"=w283, "State(s) at Back (\"\")"="UI: Uninitialize\nData: Cleanup\nExit") -> ("States Out"=w287:string)  [unwired: 13 in]
        n123 = call <vilib>:"Add State(s) to Queue__jki_lib_state_machine.vi"("State(s) in Front (\"\")"=w287, "State(s) in (\"\")"=w291) -> ("States Out"=w290:string)  [unwired: 13 in]
      }
      frame "Macro: Process Log File" {
        # "Exit Macro\n(This is called once, when the VI exits)"
        n124 = call <vilib>:"Add State(s) to Queue__jki_lib_state_machine.vi"("State(s) in Front (\"\")"="Log File: Read Data" ("State(s) in Front (\"\")"), "State(s) in (\"\")"=w296) -> ("States Out"=w295:string)  [unwired: 13 in]
      }
      frame "---------- Log File ----------" {
        # "Template Separator\n(You can make a copy of, or modify, this frame)"
        n125 = call <vilib>:"Add State(s) to Queue__jki_lib_state_machine.vi"("State(s) in (\"\")"=w300) -> ("States Out"=w299:string)  [unwired: 14 in]
      }
      frame "Log File: Read Data" {
        # "Your code here.\n(You can make a copy of, or modify, this frame)"
        n126 = Unbundle By Name(w304) -> ("log file"=w315:path)
        n127 = Open/Create/Replace File(file path (use dialog)=w315, error in=w309) -> (refnum out=w314:refnum<file>, error out=w312:errorcluster)  [unwired: 4 in, 1 out]
        n128 = Read from Text File(file (use dialog)=w314, error in=w312) -> (refnum out=w313:refnum<file>, text=w307:string, error out=w311:errorcluster)  [unwired: 2 in, 1 out]
        n129 = Close File(refnum=w313, error in=w311) -> (error out=w310:errorcluster)  [unwired: 1 out]
        n130 = call <vilib>:"Delimited String to 1D String Array.vi"("delimiter"="\n\n=*=*=*=*=*=*=*=*=*=*=*=*=*=*=*=*=*=*=*=*=*=*=*=*=*=*=*=\n", "delimited string"=w307) -> ("string array"=w306:string[])  [unwired: 9 in]
        n131 = for {
          tunnel: w306 -> [w319] mode=indexing
          tunnel: [w321] -> w302 mode=indexing if=w323
          tunnel: [w322] -> w305 mode=indexing if=w323
          tunnel: "Error Code: \"([^\"]+)\"" ("regular expression") -> [w320]
          n132 = xnode "Match Regular Expression"("input string"=w319, "regular expression"=w320) -> ("submatch 1"=w318:string)  [unwired: 4 in, 5 out]
          n133 = case shown="Default" w318 {
            selector: w318 -> [w441 _]
            tunnel: [TRUE w456] -> w323
            tunnel: [w440 w452] -> w322
            tunnel: [w445 w451] -> w321
            tunnel: w319 -> [w445 w450]
            frame Default {
              n134 = call <vilib>:"Trim Whitespace.vi"("string"=w445) -> ("trimmed string"=w446:string)  [unwired: 1 in]
              n135 = call <vilib>:"Delimited String to 1D String Array.vi"("delimiter"="\n", "delimited string"=w446) -> ("string array"=w447:string[])  [unwired: 9 in]
              n136 = Index Array(array=w447) -> (element #1=w444:string, element #2=w443:string)  [unwired: 2 in]
              n137 = Format Into String(format string="%s: %s -> %s", w444, w443, w441) -> (resulting string=w440:string)  [unwired: 2 in, 1 out]
            }
            frame "" {
              n138 = call <vilib>:"Trim Whitespace.vi"("string"=w450) -> ("trimmed string"=w458:string)  [unwired: 1 in]
              n139 = Empty String/Path?(string/path=w458) -> (empty?=w457:bool)
              n140 = call <vilib>:"Delimited String to 1D String Array.vi"("delimiter"="\n", "delimited string"=w458) -> ("string array"=w461:string[])  [unwired: 9 in]
              n141 = Not(x=w457) -> (.not. x?=w456:bool)
              n142 = Delete From Array(array=w461) -> (deleted portion=w460:string)  [unwired: 2 in, 1 out]
              n143 = Index Array(array=w461) -> (element #1=w454:string, element #2=w453:string)  [unwired: 2 in]
              n144 = Match Pattern(string=w460, regular expression=": " ("search string/char (-)")) -> (after substring=w451:string)  [unwired: 1 in, 3 out]
              n145 = Format Into String(format string="%s: %s", w454, w453) -> (resulting string=w452:string)  [unwired: 2 in, 1 out]
            }
          }
        }
        n146 = call <vilib>:"Add State(s) to Queue__jki_lib_state_machine.vi"("State(s) in (\"\")"=w317) -> ("States Out"=w316:string)  [unwired: 14 in]
        n147 = property on="timestamp" class="LstBox (strict)"("Item Names"=w305) -> ()  [unwired: 2 in, 2 out]
        n148 = Bundle By Name(cluster=w304, "elements"=w302) -> (w303:T4)
      }
      frame "New Category: 2" {
        # "Your code here.\n(You can make a copy of, or modify, this frame)"
        n149 = call <vilib>:"Add State(s) to Queue__jki_lib_state_machine.vi"("State(s) in (\"\")"=w466) -> ("States Out"=w465:string)  [unwired: 14 in]
      }
    }
  }
